vi "WaitOnStopSync.vi"(8 "error in (no error)":errorcluster, 9 "WaitForModuleToStop?":bool, 11 "ModuleAdmin":refnum<class "ModuleAdmin.lvclass">) -> (0 "error out":errorcluster, 3 "ModuleAdmin":refnum<class "ModuleAdmin.lvclass">)   [LabVIEW 2014, in "ModuleAdmin.lvlib" / "ModuleAdmin.lvclass"]
uses:
  ModuleAdmin.lvclass
  <vilib>/Utility/error.llb/Error Cluster From Error Code.vi
  <vilib>/ErrorRing/Error Ring.xnode
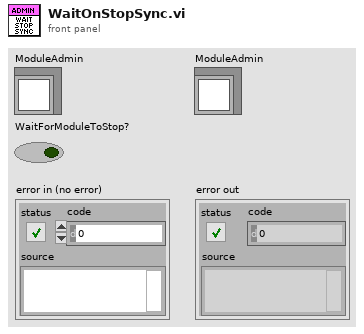
[diagram p1: front panel]
types:
  T1 = typedef "Rendezvous RefNum" = refnum<k1>
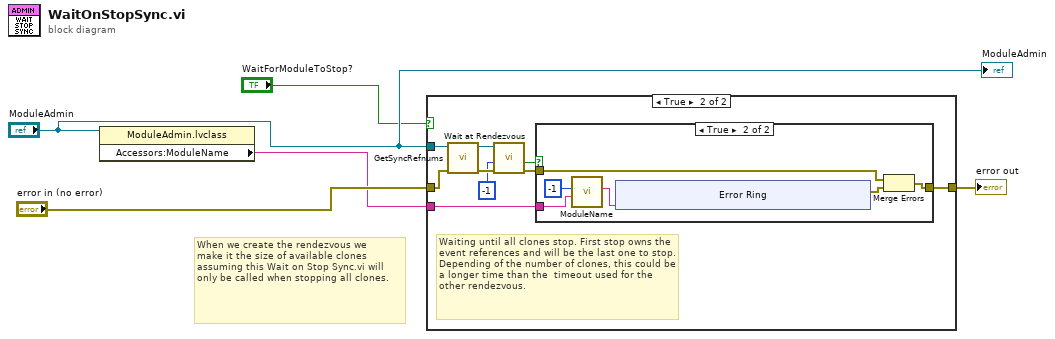
[diagram p0: block diagram]
diagram:
  # "When we create the rendezvous we\nmake it the size of available clones assuming this Wait on Stop Sync.vi will only be called when stopping all clones."
  n1 = property class="ModuleAdmin.lvclass"(reference="ModuleAdmin") -> ("Accessors:ModuleName"=w3:string)  [unwired: 1 in, 2 out]
  n2 = case shown="True" "WaitForModuleToStop?" {
    tunnel: [w6 w9] -> w4
    tunnel: "error in (no error)" -> [w6 w15]
    tunnel: w3 -> [_ w8]
    tunnel: "ModuleAdmin" -> [_ w7]
    frame False {
    }
    frame True {
      # "Waiting until all clones stop. First stop owns the event references and will be the last one to stop. Depending of the number of clones, this could be a longer time than the  timeout used for the other rendezvous."
      n3 = call "GetSyncRefnums.vi"("error in (no error)"=w15, "ModuleAdmin"=w7) -> ("error out"=w14:errorcluster, "rndzv_StopSync"=w13:T1)  [unwired: 6 in, 2 out]
      n4 = call <vilib>:"Wait at Rendezvous.vi"("error in (no error)"=w14, "ms timeout (-1)"=-1, "rendezvous"=w13) -> ("error out"=w10:errorcluster, "timed out"=w11:bool)  [unwired: 2 in, 1 out]
      n5 = case shown="True" w11 {
        tunnel: w10 -> [w16 w22]
        tunnel: [w16 w20] -> w9
        tunnel: w8 -> [_ w17]
        frame False {
        }
        frame True {
          n6 = call "ModuleName.vi"("Name"=w17, "ModuleID"=-1) -> ("ModuleName"=w18:string)  [unwired: 9 in]
          n7 = xnode "Error Ring"("parameter 0"=w18) -> ("error out"=w21:errorcluster)
          n8 = Merge Errors(w22, w21) -> (w20:errorcluster)
        }
      }
    }
  }
  "error out" <- w4
  "ModuleAdmin" <- "ModuleAdmin"
